vi "Show Caller Items Dialog.vi"(6 "Event":refnum<vi>, 8 "Find Broadcast?":bool=TRUE, 9 "Theme":bool, 11 "Request VI Callers":refnum<vi>[](array[refnum])) -> ()   [LabVIEW 2019, in "Panther Dashboard.lvlib"]
uses:
  Panther Dashboard.lvlib
  <vilib>/Utility/traverseref.llb/TRef TravTarget.ctl
  <vilib>/Utility/traverseref.llb/VI Scripting - Traverse.lvlib
panel:
  in  "View all Callers":bool
  in  "Results Listbox":i32(listbox)
  # "» Double click an element to navigate in the code\n» Right-click event to view the vi file on disk"
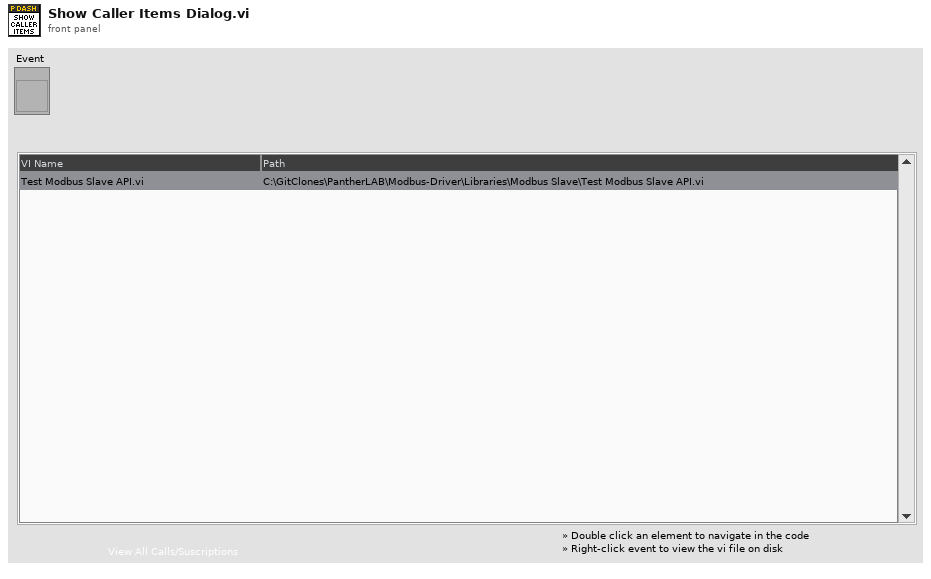
[diagram p1: front panel]
types:
  T1 = typedef "TRef TravTarget.ctl" = enum16{"FP", "BD", "Other"}
  T2 = typedef "LVRowAndColumnTypeDef.ctl" = cluster{"Row":i32, "Column":i32}
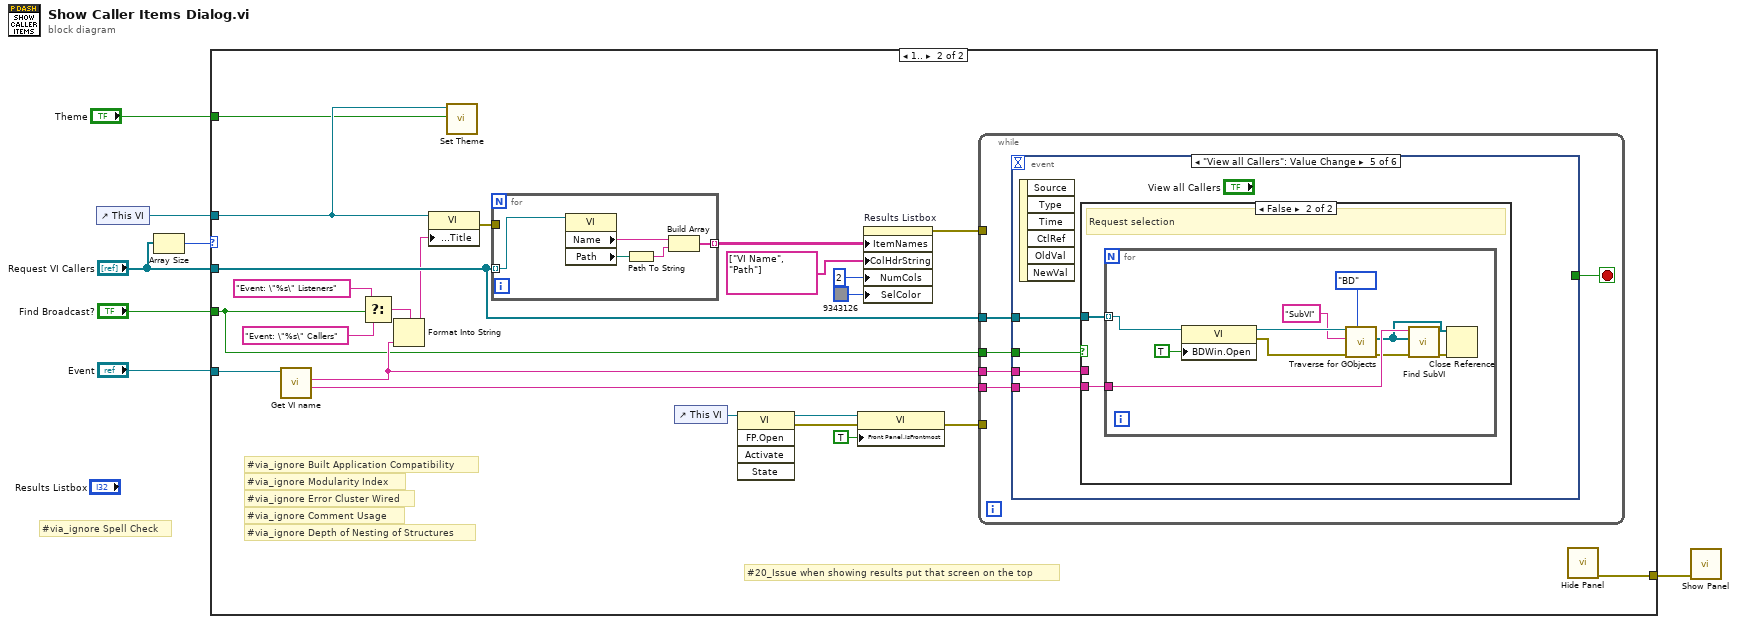
[diagram p0: block diagram]
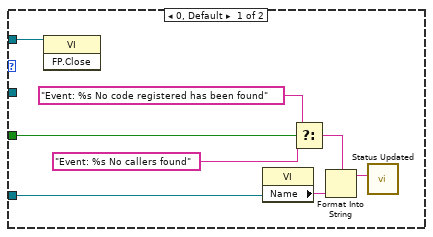
[diagram p2: hidden frame]
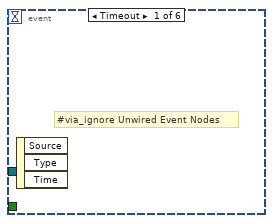
[diagram p3: hidden frame]
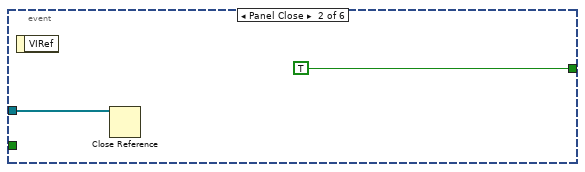
[diagram p4: hidden frame]
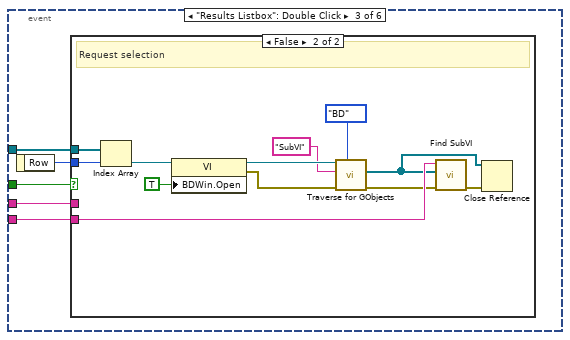
[diagram p5: hidden frame]
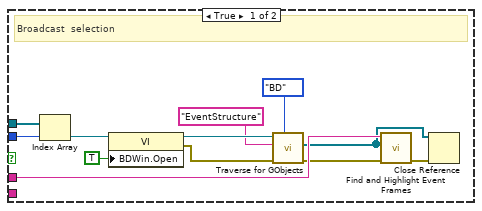
[diagram p6: hidden frame]
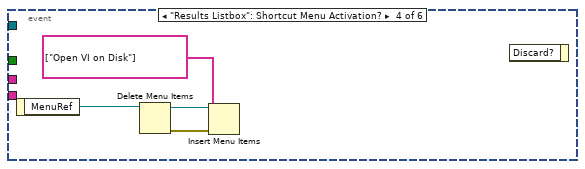
[diagram p7: hidden frame]
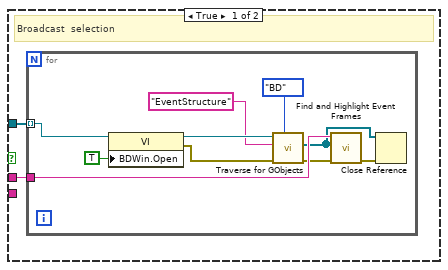
[diagram p8: hidden frame]
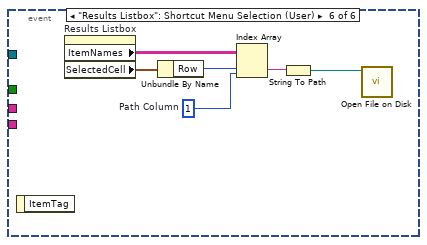
[diagram p9: hidden frame]
diagram:
  # "#via_ignore Spell Check"
  n1 = control-ref of="This VI"() -> (w2:refnum<vi>)
  n2 = Array Size(array="Request VI Callers") -> (size(s)=w6:i32)
  n3 = case shown="1.." w6 {
    tunnel: "Request VI Callers" -> [_ w30]
    tunnel: "Event" -> [w13 w28]
    tunnel: "Find Broadcast?" -> [w12 w16]
    tunnel: "Theme" -> [_ w23]
    tunnel: w2 -> [w8 w25]
    tunnel: [_ w21] -> w1
    frame 0, Default {
      n4 = invoke class="VI" method="FP.Close"(reference=w8) -> ()  [unwired: 2 in, 3 out]
      n5 = property class="VI"(reference=w13) -> ("Name"=w14:string)  [unwired: 1 in, 2 out]
      n6 = Select(t="Event: %s No code registered has been found" ("Origin"), s=w12, f="Event: %s No callers found" ("Origin")) -> (s? t:f=w10:string)
      n7 = Format Into String(format string=w10, w14) -> (resulting string=w15:string)  [unwired: 2 in, 1 out]
      n8 = call "Status Updated.vi"("Status"=w15) -> ()  [unwired: 10 in, 1 out]
    }
    frame 1.. {
      # "#20_Issue when showing results put that screen on the top"
      # "#via_ignore Built Application Compatibility"
      # "#via_ignore Modularity Index"
      # "#via_ignore Depth of Nesting of Structures"
      # "#via_ignore Error Cluster Wired"
      # "#via_ignore Comment Usage"
      n9 = call "Get VI name.vi"("VI in"=w28) -> ("Full Vi Name"=w26:string, "Plain Name"=w27:string)  [unwired: 8 in, 1 out]
      n10 = Select(t="Event: \"%s\" Listeners" ("Origin"), s=w16, f="Event: \"%s\" Callers" ("Origin")) -> (s? t:f=w32:string)
      n11 = Format Into String(format string=w32, w27) -> (resulting string=w22:string)  [unwired: 2 in, 1 out]
      n12 = property class="VI"(reference=w25, "Front Panel.Title"=w22) -> (error out=w37:errorcluster)  [unwired: 1 in, 1 out]
      n13 = call "Set Theme.vi"("Dark?"=w23, "VI in"=w25) -> ()  [unwired: 10 in]
      n14 = for {
        tunnel: w30 -> [w43] mode=indexing
        tunnel: [w39] -> w36 mode=indexing
        tunnel: w37 -> [_]
        n15 = property class="VI"(reference=w43) -> ("Name"=w42:string, "Path"=w41:path)  [unwired: 1 in, 2 out]
        n16 = Path To String(path=w41) -> (string=w40:string)
        n17 = Build Array(w42, w40) -> (w39:string[])
      }
      n18 = control-ref of="This VI"() -> (w20:refnum<vi>)
      n19 = invoke class="VI" method="FP.Open"(reference=w20) -> (reference out=w18:refnum<vi>, error out=w29:errorcluster)  [unwired: 4 in, 3 out]
      n20 = property class="VI"(reference=w18, error in=w29, "Front Panel.IsFrontmost"=TRUE ("Front Panel Window:Is Frontmost")) -> (error out=w19:errorcluster)  [unwired: 1 out]
      n21 = property on="Results Listbox" class="MCListbox (strict)"("ItemNames"=w36, "ColHdrString"=string[] ["VI Name", "Path"] ("Column Header Strings[]"), "NumCols"=u32 2 ("Number of Columns"), "SelColor"=u32 9343126) -> (error out=w38:errorcluster)  [unwired: 2 in, 1 out]
      n22 = while {
        tunnel: w30 -> [w48]
        tunnel: w38 -> [_]
        tunnel: w16 -> [w46]
        tunnel: w27 -> [w45]
        tunnel: w19 -> [_]
        tunnel: w26 -> [w44]
        stop <- w47 stop-if-true
        n23 = event shown="[4] \"View all Callers\": Value Change" {
          selector: _ -> [_ _ _ _ _ _]
          dyn-events: _ -> [_ _ _ _ _ _]
          timeout: _ -> [_ _ _ _ _ _]
          tunnel: w48 -> [_ w50 w55 _ w87 _]
          tunnel: [_ TRUE _ _ _ _] -> w47
          tunnel: w46 -> [_ _ w53 _ w84 _]
          tunnel: w45 -> [_ _ w52 _ w86 _]
          tunnel: w44 -> [_ _ w51 _ w85 _]
          event Timeout {
            # "#via_ignore Unwired Event Nodes"
            n24 = event-data() -> ()  [unwired: 1 in, 3 out]
          }
          event Panel Close {
            n25 = event-data() -> ()  [unwired: 1 in, 1 out]
            n26 = Close Reference(reference=w50) -> ()  [unwired: 1 in, 1 out]
          }
          event "Results Listbox": Double Click {
            n27 = event-data() -> ("Row"=w54:i32)  [unwired: 1 in]
            n28 = case shown="False" w53 {
              tunnel: w55 -> [w66 w78]
              tunnel: w54 -> [w65 w77]
              tunnel: w52 -> [w60 _]
              tunnel: w51 -> [_ w72]
              frame True {
                # "Broadcast  selection"
                n29 = Index Array(array=w66, index=w65) -> (element=w61:refnum<vi>)
                n30 = property class="VI"(reference=w61, "BDWin.Open"=TRUE ("Block Diagram Window:Open")) -> (reference out=w64:refnum<vi>, error out=w59:errorcluster)  [unwired: 1 in]
                n31 = call <vilib>:"Traverse for GObjects.vi"("Traverse Target"=TRef_TravTarget."BD", "error in (no error)"=w59, "Class Name"="EventStructure", "VI Refnum"=w64) -> ("error out"=w58:errorcluster, "References"=w56:refnum<vi>[])  [unwired: 4 in, 2 out]
                n32 = call "Find and Highlight Event Frames.vi"("error in"=w58, "References"=w56, "Event Name"=w60) -> ("error out"=w57:errorcluster)  [unwired: 8 in]
                n33 = Close Reference(reference=w56, error in (no error)=w57) -> ()  [unwired: 1 out]
              }
              frame False {
                # "Request selection"
                n34 = Index Array(array=w78, index=w77) -> (element=w73:refnum<vi>)
                n35 = property class="VI"(reference=w73, "BDWin.Open"=TRUE ("Block Diagram Window:Open")) -> (reference out=w76:refnum<vi>, error out=w71:errorcluster)  [unwired: 1 in]
                n36 = call <vilib>:"Traverse for GObjects.vi"("Traverse Target"=TRef_TravTarget."BD", "error in (no error)"=w71, "Class Name"="SubVI", "VI Refnum"=w76) -> ("error out"=w70:errorcluster, "References"=w68:refnum<vi>[])  [unwired: 4 in, 2 out]
                n37 = call "Find SubVI.vi"("error in"=w70, "References"=w68, "Full Vi Name"=w72) -> ("error out"=w69:errorcluster)  [unwired: 8 in]
                n38 = Close Reference(reference=w68, error in (no error)=w69) -> ()  [unwired: 1 out]
              }
            }
          }
          event "Results Listbox": Shortcut Menu Activation? {
            n39 = event-data() -> ("MenuRef"=w83:refnum<k9>)  [unwired: 1 in]
            n40 = Delete Menu Items(9:w83) -> (0:w81:errorcluster, 3:w82:refnum<k9>)  [unwired: 3 in]
            n41 = Insert Menu Items(6:w81, 8:string[] ["Open VI on Disk"] ("item names"), 9:w82) -> ()  [unwired: 3 in, 3 out]
            n42 = event-data() -> ()  [unwired: 2 in, 1 out]
          }
          event "View all Callers": Value Change {
            n43 = event-data() -> ()  [unwired: 1 in, 6 out]
            n44 = case shown="False" w84 {
              tunnel: w87 -> [w89 w101]
              tunnel: w86 -> [w88 _]
              tunnel: w85 -> [_ w100]
              frame True {
                # "Broadcast  selection"
                n45 = for {
                  tunnel: w89 -> [w92] mode=indexing
                  tunnel: w88 -> [w95]
                  n46 = property class="VI"(reference=w92, "BDWin.Open"=TRUE ("Block Diagram Window:Open")) -> (reference out=w98:refnum<vi>, error out=w94:errorcluster)  [unwired: 1 in]
                  n47 = call <vilib>:"Traverse for GObjects.vi"("Traverse Target"=TRef_TravTarget."BD", "error in (no error)"=w94, "Class Name"="EventStructure", "VI Refnum"=w98) -> ("error out"=w93:errorcluster, "References"=w90:refnum<vi>[])  [unwired: 4 in, 2 out]
                  n48 = call "Find and Highlight Event Frames.vi"("error in"=w93, "References"=w90, "Event Name"=w95) -> ("error out"=w91:errorcluster)  [unwired: 8 in]
                  n49 = Close Reference(reference=w90, error in (no error)=w91) -> ()  [unwired: 1 out]
                }
              }
              frame False {
                # "Request selection"
                n50 = for {
                  tunnel: w101 -> [w104] mode=indexing
                  tunnel: w100 -> [w107]
                  n51 = property class="VI"(reference=w104, "BDWin.Open"=TRUE ("Block Diagram Window:Open")) -> (reference out=w110:refnum<vi>, error out=w106:errorcluster)  [unwired: 1 in]
                  n52 = call <vilib>:"Traverse for GObjects.vi"("Traverse Target"=TRef_TravTarget."BD", "error in (no error)"=w106, "Class Name"="SubVI", "VI Refnum"=w110) -> ("error out"=w105:errorcluster, "References"=w102:refnum<vi>[])  [unwired: 4 in, 2 out]
                  n53 = call "Find SubVI.vi"("error in"=w105, "References"=w102, "Full Vi Name"=w107) -> ("error out"=w103:errorcluster)  [unwired: 8 in]
                  n54 = Close Reference(reference=w102, error in (no error)=w103) -> ()  [unwired: 1 out]
                }
              }
            }
          }
          event "Results Listbox": Shortcut Menu Selection (User) {
            w114 = 1  # Path Column
            n55 = event-data() -> ()  [unwired: 1 in, 1 out]
            n56 = property on="Results Listbox" class="MCListbox (strict)"() -> ("ItemNames"=w117:string[][], "SelectedCell"=w116:T2)  [unwired: 2 in, 2 out]
            n57 = Unbundle By Name(w116) -> ("Row"=w115:i32)
            n58 = Index Array(array=w117, index (row)=w115, index (col)=w114) -> (element=w113:string)
            n59 = String To Path(string=w113) -> (path=w112:path)
            n60 = call "Open File on Disk.vi"("file or directory path"=w112) -> ()  [unwired: 10 in, 1 out]
          }
        }
      }
      n61 = call "Hide Panel.vi"() -> ("error out"=w21:errorcluster)  [unwired: 11 in]
    }
  }
  n62 = call "Show Panel.vi"("error in (no error)"=w1) -> ()  [unwired: 10 in, 1 out]
